vi "Field Draw Ball.vi"(1 "element":i32, 4 "Draw Targets?":T1, 6 "balls":T2[](array[typedef]), 8 "picture in":picture, 9 "Offset":T5, 10 "Scale mm/pixel":dbl, 11 "Detection Ball":T3) -> (0 "picture out":picture)   [LabVIEW 2017]
uses:
  <vilib>/Analysis/NI_AALPro.lvlib
  <vilib>/Analysis/coordinate.llb/2D Cartesian Coordinate Rotation (Scalar).vi
  <vilib>/Utility/miscctls.llb/LVBoundsTypeDef.ctl
  SSL Detection Ball.ctl
  <vilib>/Analysis/Matrix/Datatypes/RealMatrix.ctl
  <vilib>/Analysis/Matrix/NI_Matrix.lvlib
  Core/AI Ball.ctl
  DrawTargets.ctl
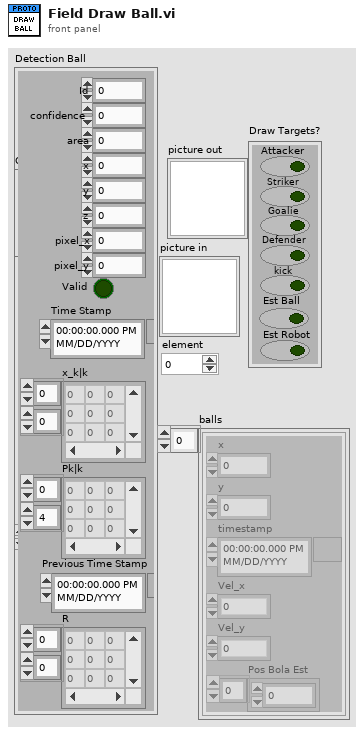
[diagram p1: front panel]
types:
  T1 = typedef "DrawTargets.ctl" = cluster{"Attacker":bool, "Striker":bool, "Goalie":bool, "Defender":bool, "kick":bool, "Est Ball":bool, "Est Robot":bool}
  T2 = typedef "AI Ball.ctl" = cluster{"x":dbl, "y":dbl, "timestamp":timestamp, "Vel_x":dbl, "Vel_y":dbl, "Pos Bola Est":dbl[]}
  T3 = typedef "SSL Detection Ball.ctl" = cluster{"x":sgl, "area":u32, "confidence":sgl, "y":sgl, "z":sgl, "pixel_x":sgl, "pixel_y":sgl, "Valid":bool, "Time Stamp":timestamp, "x_k|k":T4, "Pk|k":T4, "Id":u32, "Previous Time Stamp":timestamp, "R":T4}
  T4 = typedef "NI_Matrix.lvlib/RealMatrix.ctl" = dbl[][]
  T5 = typedef "LVBoundsTypeDef.ctl" = cluster{"Width":u32, "Height":u32}
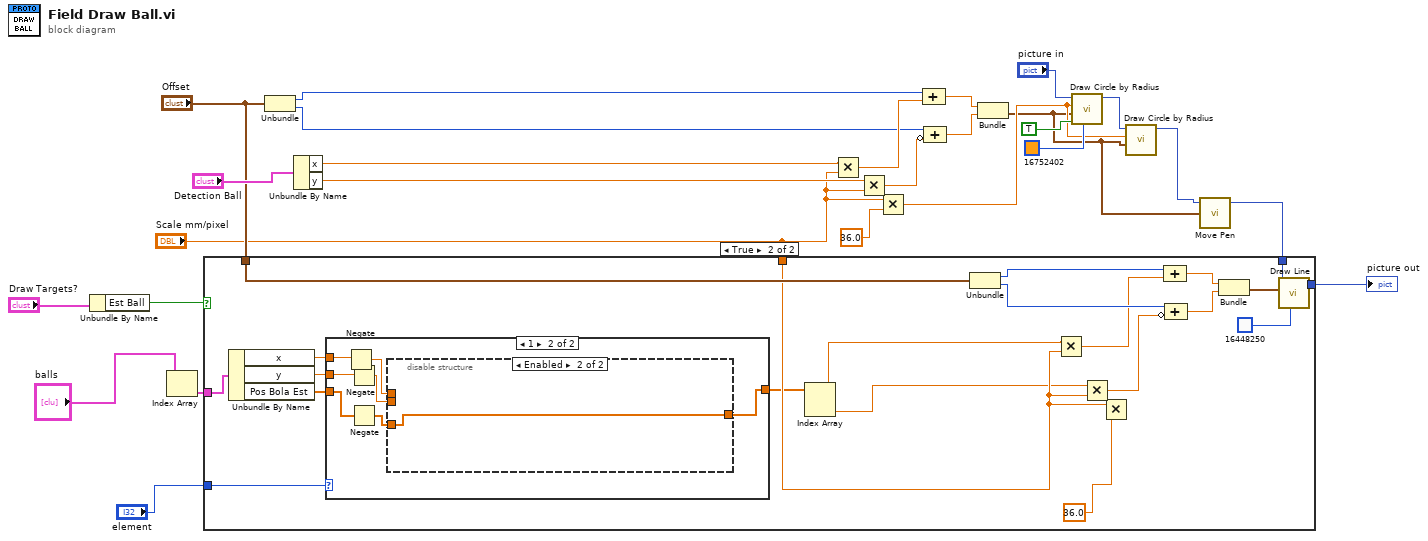
[diagram p0: block diagram]
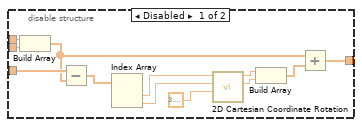
[diagram p4: hidden frame]
diagram:
  n1 = Unbundle By Name("Draw Targets?") -> ("Est Ball"=w2:bool)
  n2 = Index Array(array="balls") -> (element=w4:T2)  [unwired: 1 in]
  n3 = Unbundle("Offset") -> ("Width"=w20:u32, "Height"=w17:u32)
  n4 = Unbundle By Name("Detection Ball") -> ("x"=w22:sgl, "y"=w23:sgl)
  n5 = Multiply(x=w22, y="Scale mm/pixel") -> (x*y=w19:dbl)
  n6 = Multiply(x=w23, y="Scale mm/pixel") -> (x*y=w16:dbl)
  n7 = Multiply(x="Scale mm/pixel", y=sgl 36.0 ("radius")) -> (x*y=w12:dbl)
  n8 = Compound Arithmetic op=ADD(w20, w19) -> (w18:dbl)
  n9 = Compound Arithmetic op=ADD(w17, invert w16) -> (w15:dbl)
  n10 = Bundle(w18, w15) -> (w8:cluster{dbl, dbl})  [unwired: 1 in]
  n11 = call <vilib>:"Draw Circle by Radius.vi"("color(black)"=u32 16752402, "fill?(F)"=TRUE, "pixel center"=w8, "radius"=w12, "picture"="picture in") -> ("new picture"=w13:picture)  [unwired: 6 in]
  n12 = call <vilib>:"Draw Circle by Radius.vi"("pixel center"=w8, "radius"=w12, "picture"=w13) -> ("new picture"=w9:picture)  [unwired: 8 in]
  n13 = call <vilib>:"Move Pen.vi"("new position"=w8, "picture"=w9) -> ("new picture"=w10:picture)  [unwired: 3 in]
  n14 = case shown="True" w2 {
    tunnel: [w27 w48] -> w11
    tunnel: w10 -> [w27 w47]
    tunnel: "Offset" -> [_ w42]
    tunnel: "Scale mm/pixel" -> [_ w39]
    tunnel: w4 -> [_ w36]
    tunnel: "element" -> [_ w32]
    frame False {
    }
    frame True {
      n15 = Unbundle By Name(w36) -> ("x"=w29:dbl, "y"=w28:dbl, "Pos Bola Est"=w31:dbl[])
      n16 = case shown="1" w32 {
        tunnel: [w49 w50] -> w30
        tunnel: w31 -> [w49 w53]
        tunnel: w29 -> [_ w52]
        tunnel: w28 -> [_ w51]
        frame 0, Default {
        }
        frame 1 {
          n17 = Negate(x=w52) -> (-x=w56:dbl)
          n18 = Negate(x=w51) -> (-x=w55:dbl)
          n19 = Negate(x=w53) -> (-x=w54:dbl[])
          n20 = disable-structure shown="Enabled" {
            disable-tunnel: w56 -> [w63 _]
            disable-tunnel: w55 -> [w62 _]
            disable-tunnel: w54 -> [w61 w69]
            disable-tunnel: [w57 w69] -> w50
            frame Disabled {
              n21 = Build Array(w63, w62) -> (w58:dbl[])
              n22 = Subtract(x=w61, y=w58) -> (x-y=w60:dbl[])
              n23 = Index Array(array=w60) -> (element #1=w68:dbl, element #2=w67:dbl)  [unwired: 2 in]
              n24 = call-poly <vilib>:"2D Cartesian Coordinate Rotation.vi"("theta"=3.141592653589793, "y"=w67, "x"=w68) -> ("y out"=w65:dbl, "x out"=w66:dbl)  [unwired: 6 in, 1 out]
              n25 = Build Array(w66, w65) -> (w59:dbl[])
              n26 = Add(x=w58, y=w59) -> (x+y=w57:dbl[])
            }
            frame Enabled {
            }
          }
        }
      }
      n27 = Index Array(array=w30) -> (element #1=w35:dbl, element #2=w34:dbl)  [unwired: 2 in]
      n28 = Unbundle(w42) -> ("Width"=w46:u32, "Height"=w44:u32)
      n29 = Multiply(x=w35, y=w39) -> (x*y=w38:dbl)
      n30 = Multiply(x=w34, y=w39) -> (x*y=w37:dbl)
      n31 = Multiply(x=w39, y=sgl 36.0 ("radius")) -> ()  [unwired: 1 out]
      n32 = Compound Arithmetic op=ADD(w46, w38) -> (w45:dbl)
      n33 = Compound Arithmetic op=ADD(w44, invert w37) -> (w43:dbl)
      n34 = Bundle(w45, w43) -> (w41:cluster{dbl, dbl})  [unwired: 1 in]
      n35 = call <vilib>:"Draw Line.vi"("picture"=w47, "end point"=w41, "color(black)"=u32 16448250) -> ("new picture"=w48:picture)  [unwired: 6 in]
    }
  }
  "picture out" <- w11
